vi "set_current_image_raw.vi"(8 "error in (no error)":errorcluster, 10 "current image raw (channels)":refnum<class "Image.lvclass">[](array[class]), 11 "GenericImageProcessor.lvclass in":refnum<class "GenericImageProcessor.lvclass">) -> (0 "error out":errorcluster, 3 "GenericImageProcessor.lvclass out":refnum<class "GenericImageProcessor.lvclass">)   [LabVIEW 2010, in "GenericImageProcessor.lvclass"]
uses:
  GenericImageProcessor.lvclass
  common/classes/Image/Image/Image.lvclass
  GenericImageProcessor.lvclass/GenericImageProcessor.ctl
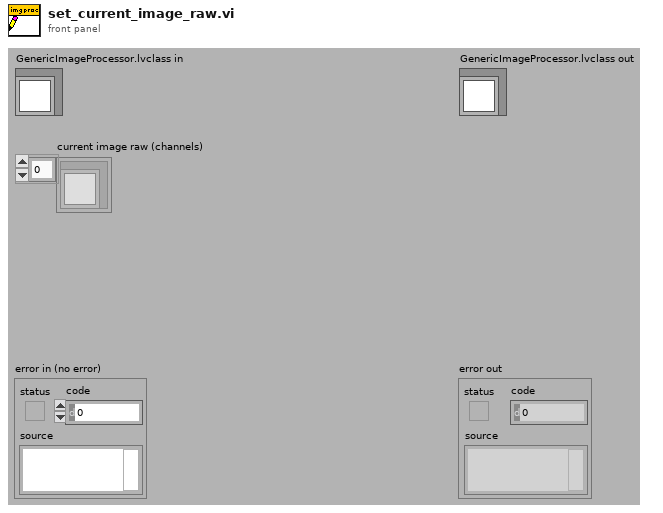
[diagram p1: front panel]
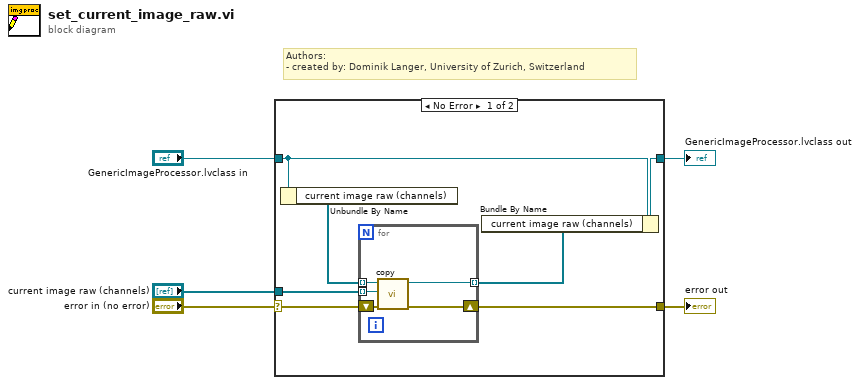
[diagram p0: block diagram]
diagram:
  # "Authors: \n- created by: Dominik Langer, University of Zurich, Switzerland"
  n1 = case shown="No Error" "error in (no error)" {
    selector: "error in (no error)" -> [w10 w18]
    tunnel: [w6 w18] -> w4
    tunnel: [w12 w19] -> w2
    tunnel: "GenericImageProcessor.lvclass in" -> [w9 w19]
    tunnel: "current image raw (channels)" -> [w11 _]
    frame No Error {
      n2 = Unbundle By Name(w9) -> ("current image raw (channels)"=w8:refnum<class "Image.lvclass">[])
      n3 = for {
        tunnel: w11 -> [w16] mode=indexing
        tunnel: w8 -> [w15] mode=indexing
        tunnel: [w14] -> w7 mode=indexing
        shift-right: [w13] -> w6
        shift-left: w10 -> [w17]
        n4 = call "copy.vi"("error in (no error)"=w17, "image to copy (source)"=w16, "Image in (target)"=w15) -> ("error out"=w13:errorcluster, "Image out"=w14:refnum<class "Image.lvclass">)  [unwired: 7 out]
      }
      n5 = Bundle By Name(cluster=w9, "current image raw (channels)"=w7) -> (w12:refnum<class "GenericImageProcessor.lvclass">)
    }
    frame Error {
    }
  }
  "error out" <- w4
  "GenericImageProcessor.lvclass out" <- w2
